vi "Run.vi"(8 "error in (no error)":errorcluster caption="entrée d'erreur (pas d'erreur)", 11 "Circles.lvclass":refnum<class "Circles.lvclass">) -> (0 "error out":errorcluster caption="sortie d'erreur", 2 "Data":T1, 3 "Circles.lvclass":refnum<class "Circles.lvclass">)   [LabVIEW 2020, in "Circles.lvclass"]
doc: "Returns : \n\nX : array of shape [n_samples, 2]\n The generated samples.\n\ny : array of shape [n_samples]\n The integer labels (0 or 1) for class membership of each sample."
uses:
  Circles.lvclass
  Circles.lvclass/Circles.ctl
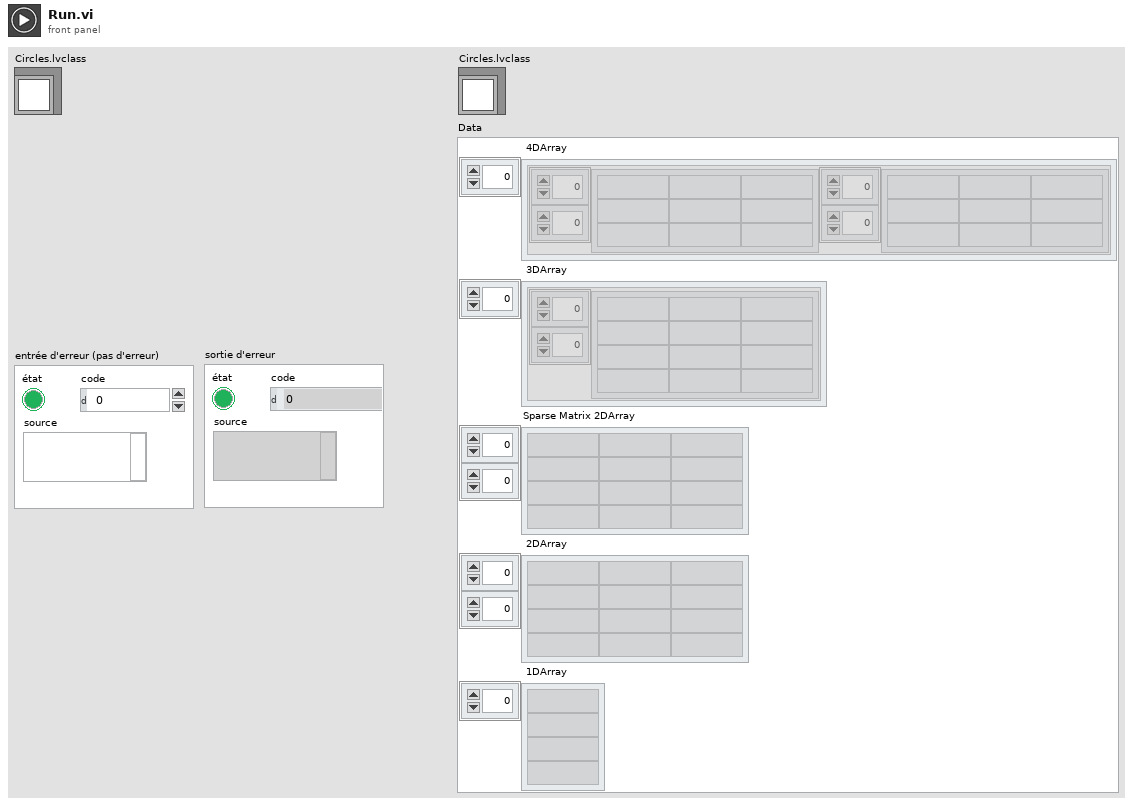
[diagram p1: front panel]
types:
  T1 = cluster{" 4DArray":cluster{"1":string[][], "2":string[][]}[], " 3DArray":cluster{"Tableau":string[][]}[], "Sparse Matrix 2DArray":string[][], " 2DArray":string[][], " 1DArray":string[]}
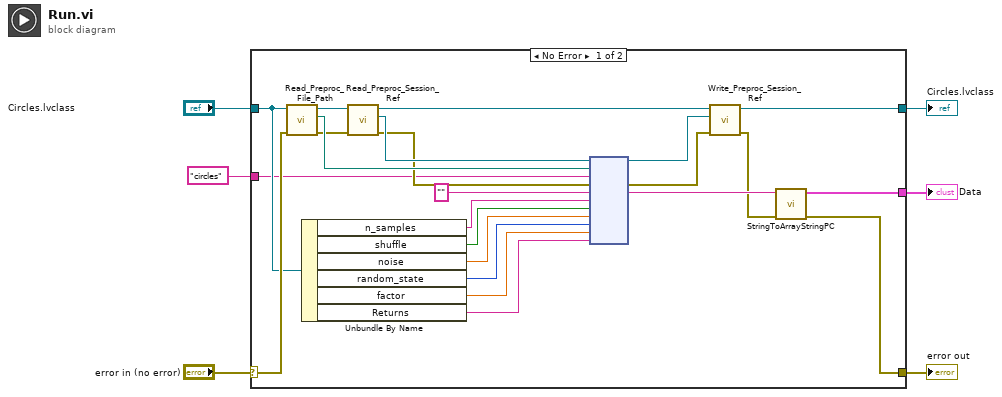
[diagram p0: block diagram]
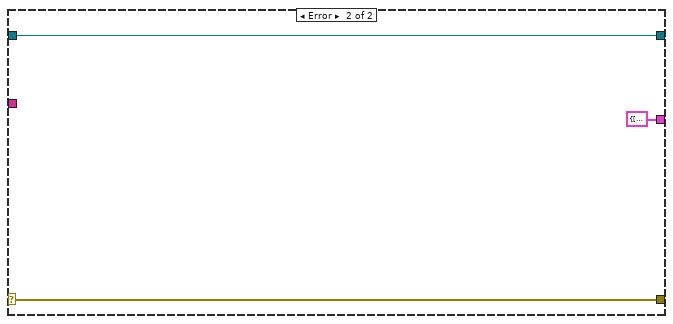
[diagram p2: hidden frame]
diagram:
  n1 = case shown="No Error" "error in (no error)" {
    selector: "error in (no error)" -> [w15 w32]
    tunnel: [w8 w32] -> w5
    tunnel: [w11 w31] -> w3
    tunnel: "Circles.lvclass" -> [w14 w31]
    tunnel: "circles" -> [w13 _]
    tunnel: [w7 T1 {" 4DArray"=[], " 3DArray"=[], "Sparse Matrix 2DArray"=[], " 2DArray"=[], " 1DArray"=[]} ("Data")] -> w1
    frame No Error {
      n2 = call-dynamic "Read_Preproc_File_Path.vi"("error in (no error)"=w15, "Python in"=w14) -> ("error out"=w24:errorcluster, "File_Path"=w27:path, "Python out"=w29:refnum<class "Circles.lvclass">)  [unwired: 7 in]
      n3 = Unbundle By Name(w14) -> ("n_samples"=w20:string, "shuffle"=w19:bool, "noise"=w18:dbl, "random_state"=w17:i32, "factor"=w16:dbl, "Returns"=w12:string)
      n4 = call-dynamic "Read_Preproc_Session_Ref.vi"("error in (no error)"=w24, "Python in"=w29) -> ("error out"=w25:errorcluster, "Session_ref"=w26:refnum<k35>, "Python out"=w28:refnum<class "Circles.lvclass">)  [unwired: 7 in]
      n5 = node(w26, w27, w13, w25, "", w20, w19, w18, w17, w16, w12) -> (w21:refnum<k35>, w23:errorcluster, w10:string)  [unwired: 6 in, 2 out]
      n6 = call-dynamic "Write_Preproc_Session_Ref.vi"("error in (no error)"=w23, "Session_ref"=w21, "Python in"=w28) -> ("error out"=w9:errorcluster, "Python out"=w11:refnum<class "Circles.lvclass">)  [unwired: 7 in]
      n7 = call "StringToArrayStringPC.vi"("sortie d'erreur"=w9, "Return value"=w10) -> ("sortie d'erreur"=w8:errorcluster, "Data"=w7:T1)  [unwired: 8 in]
    }
    frame Error {
    }
  }
  "error out" <- w5
  "Circles.lvclass" <- w3
  "Data" <- w1
